vi "go_around_left.vi"(8 "error in (no error)":errorcluster) -> (0 "error out 2":errorcluster)   [LabVIEW 2014]
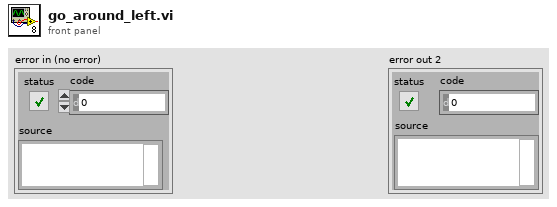
[diagram p1: front panel]
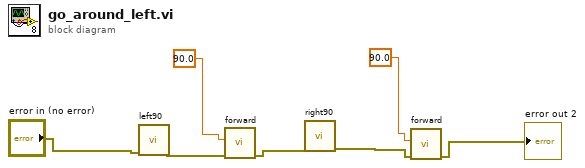
[diagram p0: block diagram]
diagram:
  n1 = call "left90.vi"("error in (no error)"="error in (no error)") -> ("error out"=w6:errorcluster)  [unwired: 9 in, 1 out]
  n2 = call "forward.vi"("error in (no error)"=w6, "Dist (cm)"=90.0) -> ("error out"=w4:errorcluster)  [unwired: 9 in]
  n3 = call "right90.vi"("error in (no error)"=w4) -> ("error out"=w3:errorcluster)  [unwired: 10 in]
  n4 = call "forward.vi"("error in (no error)"=w3, "Dist (cm)"=90.0) -> ("error out"=→"error out 2":errorcluster)  [unwired: 9 in]
